vi "Result.Measurement Look Up Limits.vi"(0 "Meas":T1 {"Status" items=["LOG", "PASS", "FAIL", "ERROR"]}, 1 "error in":errorcluster, 4 "Limits":variant) -> (5 "Measurement Out":T1 {"Status" items=["LOG", "PASS", "FAIL", "ERROR"]})   [LabVIEW 2018]
uses:
  Result.Measurement Item.ctl
  Result.Measurement and Attribute Item Status.ctl
  Result.Test Limit Item.ctl
  Result.Limit Type.ctl
panel:
  in  "Test":bool
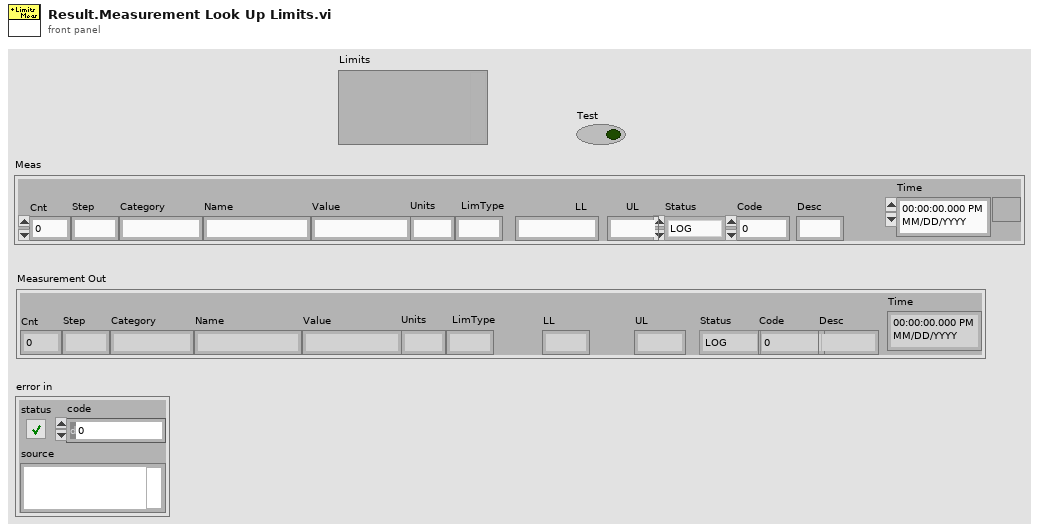
[diagram p1: front panel]
types:
  T1 = typedef "Result.Measurement Item.ctl" = cluster{"Cnt":i32, "Step":string, "Category":string, "Name":string, "Value":string, "Units":string, "LimType":string, "LL":string, "UL":string, "Status":T2, "Code":i32, "Desc":string, "Time":timestamp}
  T2 = typedef "Result.Measurement and Attribute Item Status.ctl" = i32
  T3 = typedef "Result.Test Limit Item.ctl" = cluster{"Name":string, "LimType":T4, "LL":string, "UL":string, "Units":string, "FailCode":i32, "FailDesc":string}
  T4 = typedef "Result.Limit Type.ctl" = enum16{"None", "EQ", "NE", "GT", "LT", "GE", "LE", "GTLT", "GELE", "GELT", "GTLE", "LTGT", "LEGE", "LEGT", "LTGE", "Contains", "NotContains"}
  T5 = enum16{"Time", "Error In", "Limits", "Fault Code", "Check Empty Code Desc", "Add Prefix", "Done"}
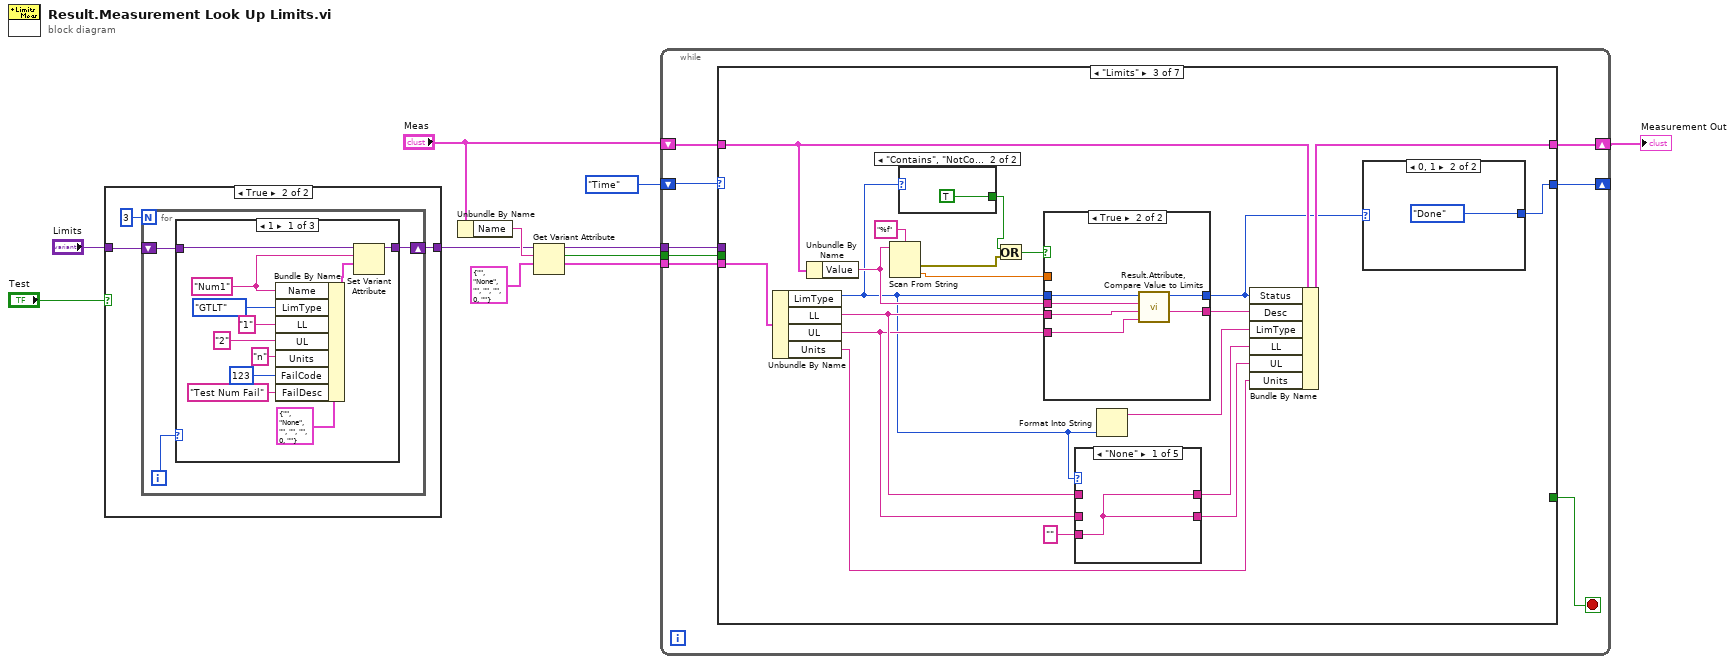
[diagram p0: block diagram]
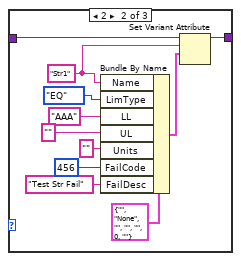
[diagram p3: hidden frame]
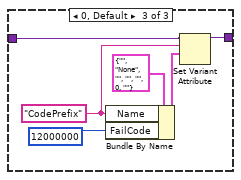
[diagram p4: hidden frame]
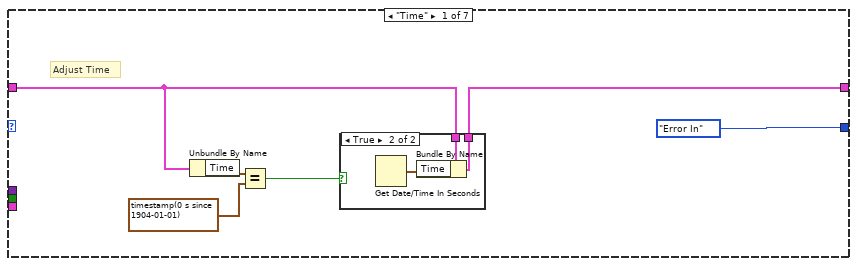
[diagram p5: hidden frame]
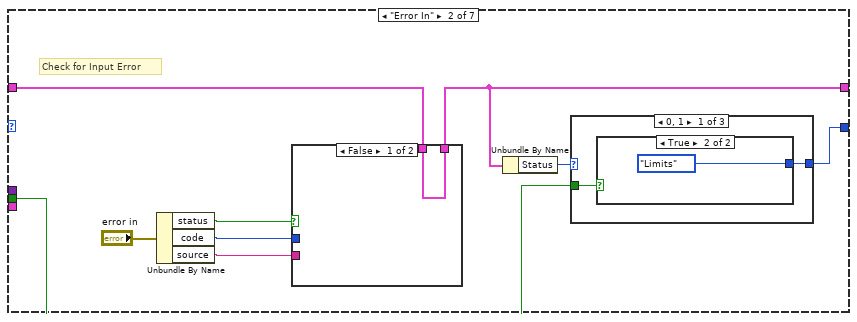
[diagram p7: hidden frame]
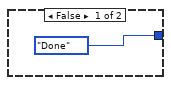
[diagram p8: hidden frame]
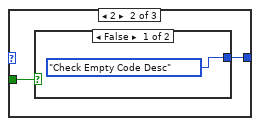
[diagram p9: hidden frame]
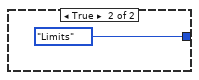
[diagram p10: hidden frame]
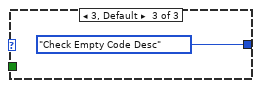
[diagram p11: hidden frame]
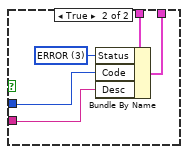
[diagram p12: hidden frame]
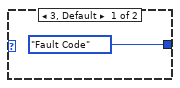
[diagram p18: hidden frame]
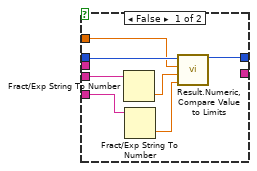
[diagram p19: hidden frame]
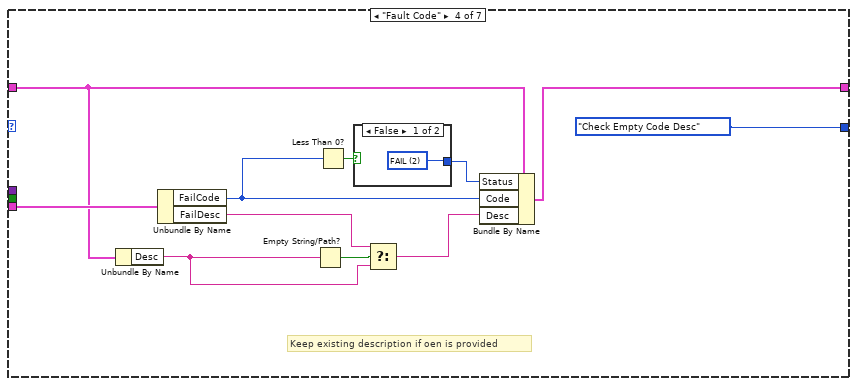
[diagram p20: hidden frame]
diagram:
  n1 = case shown="True" "Test" {
    tunnel: "Limits" -> [w12 w14]
    tunnel: [w12 w15] -> w4
    frame False {
    }
    frame True {
      n2 = for {
        N: 3 -> [_]
        shift-right: [w17] -> w15
        shift-left: w14 -> [w18]
        i -> [w16]
        n3 = case shown="1" w16 {
          tunnel: w18 -> [w21 w30 w42]
          tunnel: [w22 w31 w41] -> w17
          frame 1 {
            w20 = "Num1" ("Name")
            n4 = Bundle By Name(cluster=T3 {"Name"="", "LimType"=enum."None", "LL"="", "UL"="", "Units"="", "FailCode"=0, "FailDesc"=""} ("Result.Test Limit Item"), "Name"=w20, "LimType"=Result.Limit_Type."GTLT", "LL"="1" ("Name"), "UL"="2" ("Name"), "Units"="n", "FailCode"=123, "FailDesc"="Test Num Fail") -> (w19:T3)
            n5 = Set Variant Attribute(Variant=w21, name=w20, value=w19) -> (Variant out=w22:variant)  [unwired: 1 in, 2 out]
          }
          frame 2 {
            w39 = "Str1" ("Name")
            n6 = Bundle By Name(cluster=T3 {"Name"="", "LimType"=enum."None", "LL"="", "UL"="", "Units"="", "FailCode"=0, "FailDesc"=""} ("Result.Test Limit Item"), "Name"=w39, "LimType"=Result.Limit_Type."EQ", "LL"="AAA" ("Name"), "UL"="" ("Name"), "Units"="", "FailCode"=456, "FailDesc"="Test Str Fail") -> (w40:T3)
            n7 = Set Variant Attribute(Variant=w30, name=w39, value=w40) -> (Variant out=w31:variant)  [unwired: 1 in, 2 out]
          }
          frame 0, Default {
            w45 = "CodePrefix" ("Name")
            n8 = Bundle By Name(cluster=T3 {"Name"="", "LimType"=enum."None", "LL"="", "UL"="", "Units"="", "FailCode"=0, "FailDesc"=""} ("Result.Test Limit Item"), "Name"=w45, "FailCode"=12000000) -> (w46:T3)
            n9 = Set Variant Attribute(Variant=w42, name=w45, value=w46) -> (Variant out=w41:variant)  [unwired: 1 in, 2 out]
          }
        }
      }
    }
  }
  n10 = Unbundle By Name("Meas") -> ("Name"=w8:string)
  n11 = Get Variant Attribute(Variant=w4, name=w8, default value (empty Variant)=T3 {"Name"="", "LimType"=enum."None", "LL"="", "UL"="", "Units"="", "FailCode"=0, "FailDesc"=""} ("Result.Test Limit Item")) -> (duplicate Variant=w7:variant, found=w2:bool, value=w6:T3)  [unwired: 1 in, 1 out]
  n12 = while {
    shift-right: [w53] -> w3
    shift-left: "Meas" -> [w54]
    shift-right: [w50] -> _
    shift-left: T5."Time" -> [w51]
    tunnel: w7 -> [w49]
    tunnel: w6 -> [w48]
    tunnel: w2 -> [w47]
    stop <- w52 stop-if-true
    n13 = case shown="\"Limits\"" w51 {
      tunnel: w54 -> [w56 w69 w104 w136 w152 w167 w178]
      tunnel: [w57 w68 w103 w140 w153 w168 w178] -> w53
      tunnel: [_ _ _ _ _ _ TRUE] -> w52
      tunnel: [T5."Error In" w66 w100 T5."Check Empty Code Desc" T5."Add Prefix" T5."Done" T5."Done"] -> w50
      tunnel: w49 -> [_ _ _ _ _ w171 _]
      tunnel: w48 -> [_ _ w102 w141 _ _ _]
      tunnel: w47 -> [_ w65 _ _ _ _ _]
      frame "Time" {
        # "Adjust Time"
        n14 = Unbundle By Name(w56) -> ("Time"=w60:timestamp)
        n15 = Equal?(x=w60, y=timestamp(0 s since 1904-01-01)) -> (x = y?=w58:bool)
        n16 = case shown="True" w58 {
          tunnel: [w61 w63] -> w57
          tunnel: w56 -> [w61 w62]
          frame False {
          }
          frame True {
            n17 = Get Date/Time In Seconds() -> (seconds since 1Jan1904=w64:timestamp)
            n18 = Bundle By Name(cluster=w62, "Time"=w64) -> (w63:T1)
          }
        }
      }
      frame "Error In" {
        # "Check for Input Error"
        n19 = Unbundle By Name("error in") -> ("status"=w72:bool, "code"=w71:i32, "source"=w70:string)
        n20 = case shown="False" w72 {
          tunnel: w71 -> [_ w86]
          tunnel: w70 -> [_ w85]
          tunnel: w69 -> [w83 w88]
          tunnel: [w83 w84] -> w68
          frame False {
          }
          frame True {
            w87 = T2 3 items=["LOG", "PASS", "FAIL", "ERROR"] ("Status")
            n21 = Bundle By Name(cluster=w88, "Status"=w87, "Code"=w86, "Desc"=w85) -> (w84:T1)
          }
        }
        n22 = Unbundle By Name(w68) -> ("Status"=w67:T2)
        n23 = case shown="0, 1" w67 {
          tunnel: [w75 w79 T5."Check Empty Code Desc"] -> w66
          tunnel: w65 -> [w74 w78 _]
          frame 0, 1 {
            n24 = case shown="True" w74 {
              tunnel: [T5."Done" T5."Limits"] -> w75
              frame False {
              }
              frame True {
              }
            }
          }
          frame 2 {
            n25 = case shown="False" w78 {
              tunnel: [T5."Check Empty Code Desc" T5."Limits"] -> w79
              frame False {
              }
              frame True {
              }
            }
          }
          frame 3, Default {
          }
        }
      }
      frame "Limits" {
        n26 = Unbundle By Name(w102) -> ("LimType"=w92:T4, "LL"=w97:string, "UL"=w96:string, "Units"=w93:string)
        n27 = Unbundle By Name(w104) -> ("Value"=w106:string)
        n28 = Scan From String(format string="%f", input string=w106) -> (error out=w90:errorcluster, output 1=w105:dbl)  [unwired: 3 in, 2 out]
        n29 = case shown="\"Contains\", \"NotContains\"" w92 {
          tunnel: [_ TRUE] -> w91
          frame Default {
          }
          frame "Contains", "NotContains" {
          }
        }
        n30 = Or(x=w91, y=w90) -> (x .or. y?=w89:bool)
        n31 = case shown="True" w89 {
          tunnel: [w127 w133] -> w101
          tunnel: w92 -> [w126 w132]
          tunnel: w97 -> [w124 w131]
          tunnel: w96 -> [w123 w130]
          tunnel: [_ w129] -> w108
          tunnel: w106 -> [_ w128]
          tunnel: w105 -> [w125 _]
          frame False {
            n32 = Fract/Exp String To Number(string=w124) -> (number=w122:dbl)  [unwired: 3 in, 1 out]
            n33 = Fract/Exp String To Number(string=w123) -> (number=w121:dbl)  [unwired: 3 in, 1 out]
            n34 = call "Result.Numeric, Compare Value to Limits.vi"("UL"=w121, "LL"=w122, "Value"=w125, "LimType"=w126) -> ("Status"=w127:T2)  [unwired: 7 in]
          }
          frame True {
            n35 = call "Result.Attribute, Compare Value to Limits.vi"("UL"=w130, "LL"=w131, "Value"=w128, "LimType"=w132) -> ("Desc"=w129:string, "Status"=w133:T2)  [unwired: 6 in]
          }
        }
        n36 = case shown="\"None\"" w92 {
          tunnel: w97 -> [_ w112 w114 _ w117]
          tunnel: w96 -> [_ _ _ w115 w118]
          tunnel: "" -> [w110 w111 w113 w116 _]
          tunnel: [w110 w112 w114 w116 w117] -> w95
          tunnel: [w110 w111 w113 w115 w118] -> w94
          frame "None" {
          }
          frame "EQ".."GT", "GE" {
          }
          frame "Contains", "NotContains" {
          }
          frame "LT", "LE" {
          }
          frame Default {
          }
        }
        n37 = Format Into String(w92) -> (resulting string=w99:string)  [unwired: 3 in, 1 out]
        n38 = Bundle By Name(cluster=w104, "Status"=w101, "Desc"=w108, "LimType"=w99, "LL"=w95, "UL"=w94, "Units"=w93) -> (w103:T1)
        n39 = case shown="0, 1" w101 {
          tunnel: [T5."Fault Code" T5."Done"] -> w100
          frame 3, Default {
          }
          frame 0, 1 {
          }
        }
      }
      frame "Fault Code" {
        # "Keep existing description if oen is provided"
        n40 = Unbundle By Name(w136) -> ("Desc"=w135:string)
        n41 = Unbundle By Name(w141) -> ("FailCode"=w138:i32, "FailDesc"=w144:string)
        n42 = Empty String/Path?(string/path=w135) -> (empty?=w143:bool)
        n43 = Less Than 0?(x=w138) -> (x < 0?=w139:bool)
        n44 = case shown="False" w139 {
          tunnel: [w145 w146] -> w137
          frame False {
            w145 = T2 2 items=["LOG", "PASS", "FAIL", "ERROR"] ("Status")
          }
          frame True {
            w146 = T2 3 items=["LOG", "PASS", "FAIL", "ERROR"] ("Status")
          }
        }
        n45 = Select(t=w144, s=w143, f=w135) -> (s? t:f=w142:string)
        n46 = Bundle By Name(cluster=w136, "Status"=w137, "Code"=w138, "Desc"=w142) -> (w140:T1)
      }
      frame "Check Empty Code Desc" {
        n47 = Unbundle By Name(w152) -> ("Status"=w150:T2, "Code"=w151:i32)
        n48 = case shown="0" w151 {
          tunnel: w152 -> [w158 w162]
          tunnel: w150 -> [_ w160]
          tunnel: [w158 w159] -> w149
          frame Default {
          }
          frame 0 {
            n49 = case shown="3, Default" w160 {
              tunnel: [-5000 ("Code") 5000 ("Code")] -> w161
              frame 3, Default {
              }
              frame 2 {
              }
            }
            n50 = Bundle By Name(cluster=w162, "Code"=w161) -> (w159:T1)
          }
        }
        n51 = Unbundle By Name(w149) -> ("Desc"=w148:string)
        n52 = case shown="\"\"" w148 {
          tunnel: w149 -> [w154 w157]
          tunnel: [w154 w156] -> w153
          frame Default {
          }
          frame "" {
            n53 = Bundle By Name(cluster=w157, "Desc"="No description assigned to this failure.") -> (w156:T1)
          }
        }
      }
      frame "Add Prefix" {
        n54 = Get Variant Attribute(Variant=w171, name="CodePrefix", default value (empty Variant)=T3 {"Name"="", "LimType"=enum."None", "LL"="", "UL"="", "Units"="", "FailCode"=0, "FailDesc"=""} ("Result.Test Limit Item")) -> (value=w173:T3)  [unwired: 1 in, 3 out]
        n55 = Unbundle By Name(w173) -> ("FailCode"=w170:i32)
        n56 = Unbundle By Name(w167) -> ("Code"=w166:i32)
        n57 = Less Than 0?(x=w166) -> (x < 0?=w165:bool)
        n58 = call "TestExec.Append Fault Code Prefix.vi"("Positive(F)\\Negative(T)"=w165, "FaultCode"=w166, "FaultCode Prefix"=w170) -> ("New Fault Code"=w169:i32)  [unwired: 8 in]
        n59 = Bundle By Name(cluster=w167, "Code"=w169) -> (w168:T1)
      }
      frame "Done", Default {
      }
    }
  }
  "Measurement Out" <- w3
